vi "Winch PTO State.vi"() -> ()   [LabVIEW 2019]
panel:
  out "Engaged?":bool
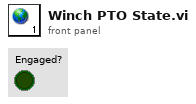
[diagram p1: front panel]
diagram:
